vi "ADCP_flush_serial_port.vi"(8 "error in (no error)":errorcluster, 11 "ADCP In":refnum<class "ADCP.lvclass">) -> (0 "error out":errorcluster, 3 "ADCP Out":refnum<class "ADCP.lvclass">)   [LabVIEW 2017, in "ADCP.lvclass"]
uses:
  ADCP.lvclass
  <vilib>/Instr/_visa.llb/VISA Flush IO Buffer Mask.ctl
  ADCP.lvclass/ADCP.ctl
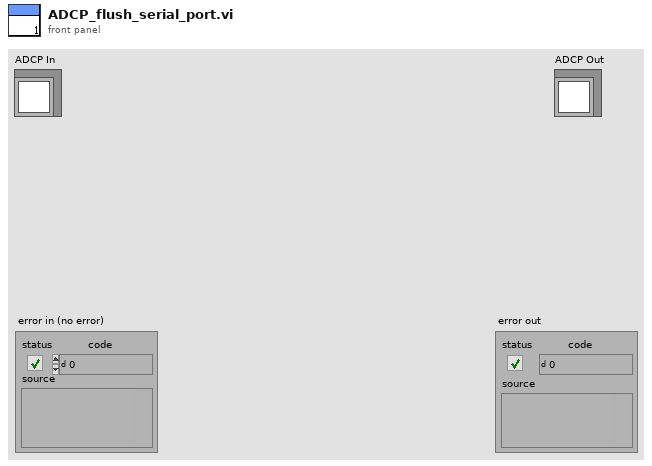
[diagram p1: front panel]
types:
  T1 = typedef "VISA Flush IO Buffer Mask.ctl" = u16
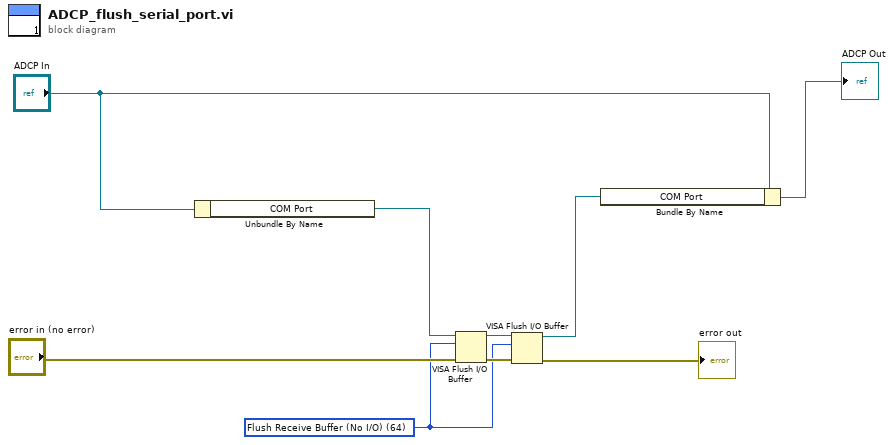
[diagram p0: block diagram]
diagram:
  w2 = T1 64 items=["Flush Receive Buffer"=16, "Write Transmit Buffer to Device"=32, "Flush Receive Buffer (No I/O)"=64, "Flush Transmit Buffer"=128] ("Mask")
  n1 = Unbundle By Name("ADCP In") -> ("COM Port"=w8:refnum<visa-resource-name>)
  n2 = VISA Flush I/O Buffer(VISA resource name=w8, mask (16)=w2, error in (no error)="error in (no error)") -> (VISA resource name out=w7:refnum<visa-resource-name>, error out=w6:errorcluster)
  n3 = VISA Flush I/O Buffer(VISA resource name=w7, mask (16)=w2, error in (no error)=w6) -> (VISA resource name out=w4:refnum<visa-resource-name>, error out=→"error out":errorcluster)
  n4 = Bundle By Name(cluster="ADCP In", "COM Port"=w4) -> (→"ADCP Out":refnum<class "ADCP.lvclass">)
